vi "SingleChannel_Plot.vi"(4 "Data column":dbl[](array[numeric]), 6 "Set voltage column":dbl[](array[numeric]), 8 "Cluster":cluster{dbl[], dbl[]}, 9 "Channel":i32, 11 "Single channel ref":refnum<vi>) -> (0 "Cluster out":cluster{dbl[], dbl[]})   [LabVIEW 2016]
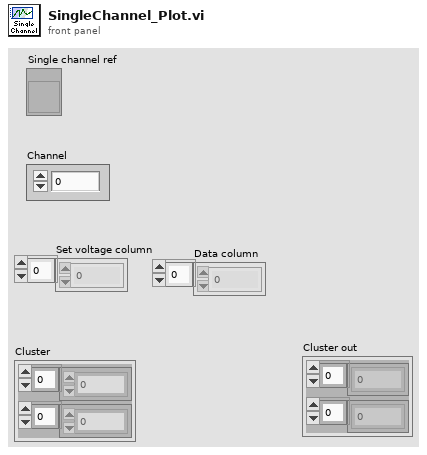
[diagram p1: front panel]
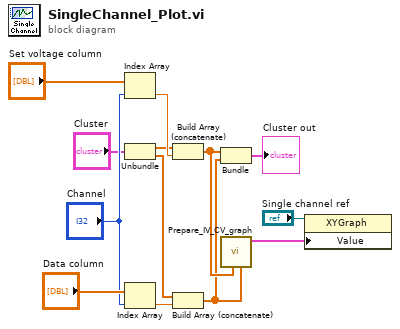
[diagram p0: block diagram]
diagram:
  n1 = Index Array(array="Set voltage column", index="Channel") -> (element=w13:dbl)
  n2 = Unbundle("Cluster") -> (w5:dbl[], w4:dbl[])
  n3 = Index Array(array="Data column", index="Channel") -> (element=w12:dbl)
  n4 = Build Array (concatenate)(w5, w13) -> (w3:dbl[])
  n5 = Build Array (concatenate)(w4, w12) -> (w2:dbl[])
  n6 = Bundle(w3, w2) -> (→"Cluster out":cluster{dbl[], dbl[]})  [unwired: 1 in]
  n7 = call "Prepare_IV_CV_graph.vi"("Y array"=w2, "X array"=w3) -> ("XY Graph"=w11:cluster{"X array":dbl[], "Y array":dbl[]}[])  [unwired: 9 in]
  n8 = property class="XYGraph"(reference="Single channel ref", "Value"=w11) -> ()  [unwired: 1 in, 2 out]
